vi "observacao_queued.vi"() -> ()   [LabVIEW 2012, in "Shared_160.lvlib"]
uses:
  Shared_160.lvlib
  Control 1.ctl
  System.Windows.Forms
  Global_Telescopio.vi
  Global Tabs.vi
panel:
  out "element":string
  out "size(s)":i32
  out "timeStatShutterAlert":i32
  out "sendCommandShutter":bool
  out "shutterTimeOld":i32
  out "LEAF":i32
  in  "Default":string="DEFAULT"
  out "Flag ativo DEC":bool
  out "Flag ativo AH":bool
  out "Flag de erro p/ apagar lampada":bool
  out "Cont-ShutOpen":timestamp
  out "Flag-ShutClose":bool
  out "Flag-ShutOpen":bool
  in  "erro lig":i32=3
  in  "erro des":i32=3
  in  "xxz":string
  out "Flag desligar":bool
  out "Flag ligar":bool
  out "Flag Stop":bool
  in  "AUX LAMPADA":bool
  out "Apontou":bool caption="Working Area"
  in  "AUX ABA":bool
  out "error out 5":errorcluster
  in  "error in (no error)":errorcluster
  out "AH_Destino":dbl format="%.9g"
  out "CONT DEC UTILS":i32
  out "CR DEC UTILS":i32
  out "CONT AH UTILS":i32
  out "CR AH UTILS":i32
  out "Erro PROTEC":i32=5
  out "Erro Lim":i32=5
  out "Flag Alarm":bool
  out "alarm Time":timestamp
  out "error out 4":errorcluster
  in  "Case Constant\n(See Context Help) 21":bool=TRUE
  in  "Case Constant\n(See Context Help) 19":bool=TRUE
  in  "Case Constant\n(See Context Help) 18":bool
  in  "Case Constant\n(See Context Help) 17":bool=TRUE
  in  "Case Constant\n(See Context Help) 16":bool
  in  "LedPointing":bool=TRUE
  in  "Case Constant\n(See Context Help) 15":bool
  in  "Case Constant\n(See Context Help) 14":bool=TRUE
  in  "Case Constant\n(See Context Help) 13":bool=TRUE
  in  "Case Constant\n(See Context Help) 12":bool=TRUE
  in  "Case Constant\n(See Context Help) 11":bool
  in  "Case Constant\n(See Context Help) 10":bool
  in  "Case Constant\n(See Context Help) 9":bool
  in  "Disabled":u8=2
  in  "Case Constant\n(See Context Help) 8":bool=TRUE
  in  "Case Constant\n(See Context Help) 7":bool=TRUE
  in  "Case Constant\n(See Context Help) 6":bool
  in  "Case Constant\n(See Context Help) 5":bool
  in  "TRUE=HORA\nFALSE=GRAU":bool=TRUE
  in  "Case Constant\n(See Context Help) 4":bool
  in  "Case Constant\n(See Context Help) 3":bool
  in  "Case Constant\n(See Context Help) 2":bool
  in  "Case Constant\n(See Context Help)":bool
  out "TA3":u32
  out "TA2":u32
  out "TF2":u32
  out "TF1":u32
  out "TA1":u32
  out "Tick Cupula":u32
  out "T2 3":u32
  in  "ESTADO ABRIR":string
  in  "ESTADO FECHAR":string
  out "T2 2":u32
  out "T1 2":u32
  out "T2":u32
  out "T1":u32
  out "DEC":string="00 00 00,00"
  out "Hour Angle 2":string="00 00 0,00" caption="AH"
  in  "TIMER TICK":u32
  in  "STOP":bool
  in  "News":bool
  out "AtmosferaStr":string
  in  "BtShutterClose":bool caption="DOME SHUTTER"
  out "HA obs":dbl
  out "Time to Limit":string
  in  "Clear All Messages":bool
  out "FiltroDuplo":bool
  out "ObjCentrado":bool
  out "Timeout PROT":u32
  out "LIMITE":bool
  in  "DestCUP":i16
  in  "DestAH":dbl
  in  "DestDEC":dbl
  in  "M_CUP":i32
  out "TimeoutCUP 2":u32
  out "TimeoutAH 2":u32
  out "TimeoutDEC 2":u32
  in  "Max":dbl=2300.0
  in  "Min":dbl=200.0
  out "error out":errorcluster
  out "TUBO_STAT":string
  out "CUP_STAT":string
  out "DEC_STAT":string
  out "AH_STAT":string
  out "FOCO_ENC":string
  out "DEC_ENC":string
  out "AH_ENC":string
  out "RA on Target":bool
  in  "BtOnTatget":bool
  out "Offset DEC":dbl format="%#.2f"
  out "Offset RA":dbl format="%#.2f"
  out "Mount Fine Movement":bool
  out "Mount Gross Movement":bool
  in  "follow redirects (T)":bool=TRUE
  out "header":string
  out "subarray":string[][](array[string])
  out "Draw Area 4":cluster{"Width":u32, "Height":u32}
  out "Draw Area 3":cluster{"Width":u32, "Height":u32}
  in  "sair":bool
  out "Saida Path string":string
  out "AUX EDITA RA":string caption="Name"
  out "Sideral time":string caption="ST"
  out "UT":string
  out "FLAG SET COORD":bool
  out "AUX EDITA PMDEC":string caption="Name"
  out "AUX EDITA PMRA":string caption="Name"
  out "AUX EDITA EPOCH":string caption="Name"
  out "AUX EDITA DEC":string caption="Name"
  out "AUX EDITA Name":string caption="Name"
  out "Hour Angle":string="00 00 0,00"
  in  "DECTARGET":string
  in  "AHTARGET":string
  out "Zenital angle":dbl
  out "SlideEnviromental":dbl(slide) caption="Progress ..." scale=0.0..100.0
  out "RA AUX":string
  out "EPOCH AUX":string
  out "Draw Area 2":cluster{"Width":u32, "Height":u32}
  out "SYSTEM MESSAGES":string
  out "Data Acquisition Activity":bool
  out "Auto guider Activity":bool
  out "Security Zone":bool
  out "Precess Data out-of-date":bool
  out "D...":bool
  out "C...":bool
  out "B...":bool
  out "A...":bool
  out "DEC on Target":bool
  out "Dome on Target":bool
  out "Remote User in Control":bool
  out "Air Mass":dbl
  out "Epoch":dbl
  out "Right Ascention":string="00 00 00,00"
  out "Declination":string="00 00 00,00"
  out "Azimuth":dbl
  out "Wind Chill":dbl
  out "Boolean 11":bool
  out "Wind Dir":string
  in  "Int/Ext":bool=TRUE
  out "Temperature":dbl
  out "Humidity":dbl
  out "Dew Point":dbl
  out "Wind Speed":dbl
  out "Pressure":dbl
  in  "RESTART METEOR":bool
  in  "VARIABLE \nTRACKING":bool
  out "LED VAR TRACKING":bool
  out "LED GUIDER":bool
  out "Led Chave Dome":bool
  out "LED MOUNT":bool
  in  "GUIDER":bool
  in  "DOME":bool
  in  "MOUNT":bool
  out "NAME":string
  out "DEC":string
  out "RA":string
  in  "Tab Control":T1(tab)=enum."Test Only"
  in  "IMAGE 5":bool
  out "Image":picture
  in  "PictureBox":refnum<k24>(container)
  out "Image 2":picture
  in  "IMAGE 2":bool
  out "error out 3":errorcluster
  out "error out 2":errorcluster
  in  "IMAGE 4":bool
  out "Image 4":picture
  out "pressão atm":string
  out "hum local":string
  out "Temp amb":string
  in  "IMAGE 3":bool
  out "Image 3":picture
  in  "IMAGE 6":bool
  out "Image 3a":picture
  out "C. AH":i32
  out "DOMO_ENC":string
  out "Proteção":bool
  in  "M_PROT":i32
  out "dt":u32
  out "TUBO":bool[](array[boolean])
  out "CUP":bool[](array[boolean])
  out "DEC":bool[](array[boolean])
  out "RA":bool[](array[boolean])
  in  "statCUP":i32
  in  "statAH":i32
  in  "statDEC":i32
  out "statCUP 2":i32
  out "TimeoutCUP":u32
  out "Azimute cup":u16
  out "PosCUP":i16
  out "dtAUX2":u32
  out "dtAUX3":u32
  out "PosAH":dbl
  out "PosDEC":dbl
  out "dec=":bool
  out "ah=":bool
  in  "CR AH":i32
  in  "CR DEC":i32
  out "C. DEC":i32
  in  "M_AH":i32
  in  "M_DEC":i32
  in  "Stop All":bool
  in  "Setup, Pointing & Guiding":T2(tab)=enum."POINTING"
  in  "RA Max 2":i32 min=-6 max=23
  in  "RA Min 2":i32 min=-6 max=23
  out "Erro":bool
  in  "MAG Max":dbl min=-9.0 max=100.0
  in  "MAG Min":dbl min=-9.0 max=25.0
  in  "DEC Max":i32 min=-90 max=90
  in  "DEC Min":i32 min=-90 max=90
  in  "RA Max":i32 caption="AH Max" min=-6 max=23
  in  "RA Min":i32 caption="AH Min" min=-6 max=23
  in  "Filter RA":bool
  in  "Slide old":i32
  out "Tot Linhas":i32
  in  "Open BSC":bool
  in  "Slide":dbl(slide) min=0.0 max=24.0 step=0.024 scale format="%#_3g"
  in  "EDIT":bool
  in  "Insert":bool
  out "List File":string
  in  "Upload":bool
  in  "Open":bool
  in  "Save AS":bool
  in  "Save":bool
  in  "Clear ALL":bool
  in  "SET coord":bool
  in  "Delete":bool
  in  "Multicolumn Listbox":i32[](listbox)
  out "ScaleMin":string
  out "ScaleMax":string
  out "DEC obs":dbl format="%.9f"
  out "RA obs":dbl format="%.9f"
  in  "ChkPointPrecessed":bool
  in  "Processa Centragem":bool
  out "PM_DEC":string
  out "PM_RA":string
  out "LedPointing":bool caption="Telescope Pointing"
  out "TimeoutAH":u32
  out "TimeoutDEC":u32
  out "AtualDEC":dbl format="%.9f"
  out "MeanDEC":string
  out "MeanRA":string
  in  "MAG":string
  out "Zenital Angle":string
  out "Air Mass":string
  out "Tempo Obs":string
  in  "BtPointPrecess":bool
  in  "ChkCalGlobal":bool=TRUE
  in  "ChkCalLocal":bool caption="Use Local Zero"
  in  "ChkPoinLampOFF":bool=TRUE
  in  "ChkPointRNA":bool
  in  "ChkModel":bool=TRUE
  in  "ChkWindDown":bool
  in  "ChkOpenShutter":bool
  in  "ChkDomeEnable":bool
  out "LedPointWorkArea":bool caption="Working Area"
  in  "BtTargetPoint":bool
  out "StrPointTargetDEC":string caption="Declination"
  out "StrPointTargetRA":string caption="Right Ascension"
  in  "BtPointObjClear":bool
  in  "StrPointObjPMDEC":string caption="DEC Proper Motion"
  in  "StrPointObjPMRA":string caption="RA Proper Motion"
  in  "StrPointObjName":string caption="Name"
  in  "StrPointObjEpoch":string caption="Epoch"
  in  "StrPointObjDEC":string caption="Declination"
  in  "StrPointObjRA":string caption="Right Ascension"
  out "MOV_IDX_DEC":bool
  out "MOV_IDX_AH":bool
  out "LatchDeslocDEC":dbl caption="DEC"
  out "LatchDeslocRA":dbl caption="RA"
  in  "ClearDeslocDEC":bool
  in  "ClearDeslocRA":bool
  out "DeslocDEC":dbl caption="DEC" format="%#.1f"
  out "DeslocRA":dbl caption="RA" format="%#.1f"
  in  "Delete Calagem":bool
  in  "Global":bool caption="Local"
  in  "Calagem":bool
  in  "Up HS":bool
  in  "Right HS":bool
  in  "Down HS":bool
  in  "Left HS":bool
  in  "Velocity (arcsec/sec)":i32(slide) min=0 max=600 scale=0.0..600.0
  in  "BtPrecGO":bool
  in  "BtPrecCentrar":bool
  in  "PreciseOffsetDEC":dbl caption="DEC" min=-10000.0 max=10000.0 step=1.0 format="%.3g"
  in  "PreciseOffsetRA":dbl caption="RA . cos(delta)" min=-10000.0 max=10000.0 step=1.0 format="%.3g"
  in  "Habilita Movimento":bool=TRUE
  in  "Y STAR":i32=1 min=1 max=400 step=1
  in  "X STAR":i32=1 min=1 max=400 step=1
  in  "XY CENTER":bool
  in  "Y CENTER":i32=1 min=1 max=400 step=1
  in  "X CENTER":i32=1 min=1 max=400 step=1
  in  "ClearRA":bool
  in  "ClearDEC":bool
  in  "DEC RATE":i32 min=-2000 max=2000 step=1
  in  "RA  RATE":i32 min=-2000 max=2000 step=1
  out "old":i32 min=0 max=360
  in  "Velocity":dbl(slide)=0.01 caption="(max = 65535 u/s)" min=0.01 max=100.0 step=0.01 scale=0.0..100.0
  in  "focusHome":bool
  out "focusStatus":string="            Focus Status"
  out "focuAlarm":bool caption="Motor temp."
  out "focusHoming":bool caption="Homing"
  out "focusMoving":bool caption="Moving"
  out "focusConnected":bool
  out "focusInitialized":bool
  in  "SetDefaultFocus":bool
  out "Foco":dbl(slide) caption="1" scale=0.0..50000.0
  in  "Setpoint":dbl=200.0 caption="Target" min=200.0 max=2300.0 step=1.0
  in  "GO":bool
  in  "Focus +":bool caption="Focus Out (+)"
  in  "Focus -":bool caption="Focus In (-)"
  in  "New Angle":string="    0.0"
  out "Default Angle":string="      0.00"
  in  "SetRotatorDefAngle":bool
  in  "Set Rotator Angle":bool
  out "Rotator Angle":string="  0.00" caption="for  GUIDING"
  out "StatShutterFile":string
  out "Command":string
  in  "CCW":bool
  out "RefreshShutterState":bool
  in  "BtParavStop":bool
  in  "BtParavUp":bool
  in  "BtParavDown":bool
  out "LedShutter":bool
  out "TimeoutTrap":u32
  out "StatShutter":string caption="Control State"
  in  "BtShutClose":bool
  in  "BtShutOpen":bool
  out "StatDome":string caption="Control State"
  in  "BtDomeSTOP":bool
  in  "BtDomeGO":bool caption="DOME"
  in  "DomeNewPos":i32=30 caption="New Position" min=0 max=360
  out "PosCup":i16 caption="Position"
  in  "CW":bool
  out "LED ACTION":bool
  out "LED MODE":bool
  in  "ACTION":bool
  in  "MODE":bool
  in  "Default Met":bool=TRUE
  in  "PROTEÇÃO":bool
  in  "STOP":bool
  in  "Enable Centragem":bool=TRUE
  in  "GO":bool
  in  "StrPointObjDEC 2":string caption="DEC"
  in  "StrPointObjRA 2":string caption="AH"
  out "MOVING":bool
  in  "FLAT-FIELD":bool
  in  "BtUtilPark":bool
  in  "ECASS":bool
  in  "BtUtilZenith":bool
  in  "TabInstrumento":T3(tab)=enum."Cam 1"
  out "Posição Rede":i32=10 caption="Largura da Fenda" min=10 max=5000 step=1
  in  "HomePrisma":T4 caption="DOME"
  in  "HomeEspelho":T4 caption="DOME"
  in  "HomeFenda":T4 caption="DOME"
  in  "IronArc":bool=TRUE
  out "Boolean":bool
  out "Largura da Fenda 2":dbl=10.0 caption="Largura da Fenda" min=10.0 max=5000.0 step=1.0
  in  "Prisma das Lâmpadas":bool
  out "Position":string
  in  "Largura da Fenda":dbl=10.0 min=10.0 max=5000.0 step=1.0
  in  "Go Largura da Fenda":bool caption="DOME"
  in  "Angulo da rede de difração":i32=10 caption="Ângulo da Rede" min=10 max=99989 step=1
  in  "Go Angulo de Difração":bool caption="DOME"
  in  "Incand":bool=TRUE
  in  "Neon":bool=TRUE
  in  "Cathode":bool=TRUE
  out "Ang. Fenda":dbl
  in  "Go_Coudé":bool
  in  "Radio Buttons":enum32{"Azul", "Visível", "Vermelho"}(radio)
  out "EndTime":u32
  out "ledAzul":bool
  out "ledVisivel":bool
  out "ledVermelho":bool
  in  "MENSAGEM":string="EM MOVIMENTO"
  out "MENSAGEM 2":string="EM MOVIMENTO"
  out "#2":bool
  out "#3":bool
  out "#4":bool
  out "PosSecundario":bool
  out "Cjto_3":bool
  out "EspAtual":string
  out "parou":bool
  out "parou 2":bool
  out "Posição Espelho":dbl=10.0 caption="Largura da Fenda" min=10.0 max=5000.0 step=1.0
  out "parou 3":bool
  out "Output Message":string
  in  "stopEcass":bool
  out "SlideEcass":u8(slide) caption="Espelho movendo..." max=100 scale=0.0..100.0
  out "LedRep":bool
  out "LedCal":bool
  in  "Sent_EspLampCass":bool
  out "LedHe":bool
  out "LedNe":bool
  in  "He-Ar":bool
  in  "Ne":bool
  in  "stopCam1":bool
  out "SlideCam1":u8(slide) caption="Espelho movendo..." max=100 scale=0.0..100.0
  out "LedRepCam1":bool
  out "LedCalCam1":bool
  in  "Sent_EspDesvFeixe":bool
  in  "Go_filtro":bool
  in  "Filtro":string(combo)
  in  "Mover/Parar":bool
  out "Recuar":bool
  in  "Sentido":bool=TRUE
  in  "Velocidade":bool
  out "Rapido":bool
  out "Lento":bool
  out "Avancar":bool
  out "Comando":string
  in  "Mensage Alarme":string="To light up close the Shutter !"
  out "CoudeSel":bool
  in  "Coude":bool
  in  "BtCalFlatField":bool
  in  "ChkCalLamp4":bool
  in  "ChkCalLamp3":bool
  in  "ChkCalLamp2":bool
  in  "ChkCalLamp1":bool
  in  "BtCalTurnOff":bool
  in  "BtCalTurnOn":bool
  out "StrongSel":bool
  out "MediumSel":bool
  out "WeakSel":bool
  in  "Strong":bool
  in  "Medium":bool
  in  "Weak":bool
  # "TELESCOPE CONTROL SYSTEM\nPICO DOS DIAS OBSERVATORY"
  # "Status Information"
  # "System Positions"
  # "Environmental Status"
  # "EXT"
  # "INT"
  # "mBar"
  # "o"
  # "C"
  # "Km/h"
  # "%"
  # "o"
  # "o"
  # "C"
  # "C"
  # "CLOUSURE LIMITS"
  # "Wind Speed            >  70 Km/h\nRelative Humidity    >  97 %\nInternal Dewpoint  <  0.5  C\nExternal Dewpoint <  1.0  C"
  # "OBJECT"
  # "TRACKING ENABLE"
  # "%"
  # "Conector 4"
  # "Conector 3"
  # "ALARME\nATENÇÃO\nERROS\nOCUPADO"
  # "Proteção\n\nTracking\nVar_Track"
  # "Rapido\nLigeiro\nFino\nRun"
  # "Motor\nIDX_Rdy\nManual"
  # "BSC FILTERS"
  # "LIST FILE"
  # "OBJECT INPUT"
  # "TARGET"
  # "OPTIONS"
  # "MANUAL OFFSET"
  # "PRECISE OFFSET"
  # "N"
  # "E"
  # "W"
  # "arcsec"
  # "arcsec"
  # "S"
  # "DISPLACEMENT"
  # "CALAGEM"
  # "PODE NÃO FUNCIONAR CORRETAMENTE!"
  # "STAR CENTERING"
  # "VAR. TRACKING"
  # "AUTO-GUIDER COORDINATES"
  # "1) Entrar X e Y do cursor do Autoguider correspondente à posição de centragem nas entradas X CENTER e Y CENTER. \n2) Após apontamento, entrar em X STAR e Y STAR os valores de X e Y do Autoguider com o \"Guide Box\" sobre o objeto apontado. \n3) Clicar em MOVE STAR TO CENTER."
  # "May take many\ntens of seconds"
  # "(instrument)"
  # "Continuous Movement"
  # "ATENÇÃO:\nO Rotator ainda não está integrado ao sistema de controle e como sua posição afeta a guiagem, sempre que o rotator for girado manualmente é necessário digitar o valor de sua nova posição no controle \"New Angle\" e pressionar \"SET NEW\".\n\nPressionar \"SET NEW\" ou \"SET DEFAULT\" não gira o rotator!"
  # "ROTATION"
  # "SHUTTER"
  # "WINDSCREEN"
  # "Covers"
  # "FIXED POSITIONS"
  # "Acquisition System\nON TARGET command"
  # "Select one Mirrror"
  # "Mirror #2"
  # "Mirror #3"
  # "Mirrors Drivers"
  # "Lâmpadas de Calibração"
  # "Espelho das Lâmpadas de Calibração"
  # "Posição"
  # "Repouso"
  # "Ativo"
  # "LIGA"
  # "LIGA"
  # "DESL."
  # "DESL."
  # "Espelho do Eucalyptus"
  # "Roda de filtros"
  # "Posição"
  # "Repouso"
  # "Ativo"
  # "Espelho de Campo"
  # "Recuar"
  # "Avançar"
  # "Rápido"
  # "Lento"
  # "CALIBRATION LAMPS"
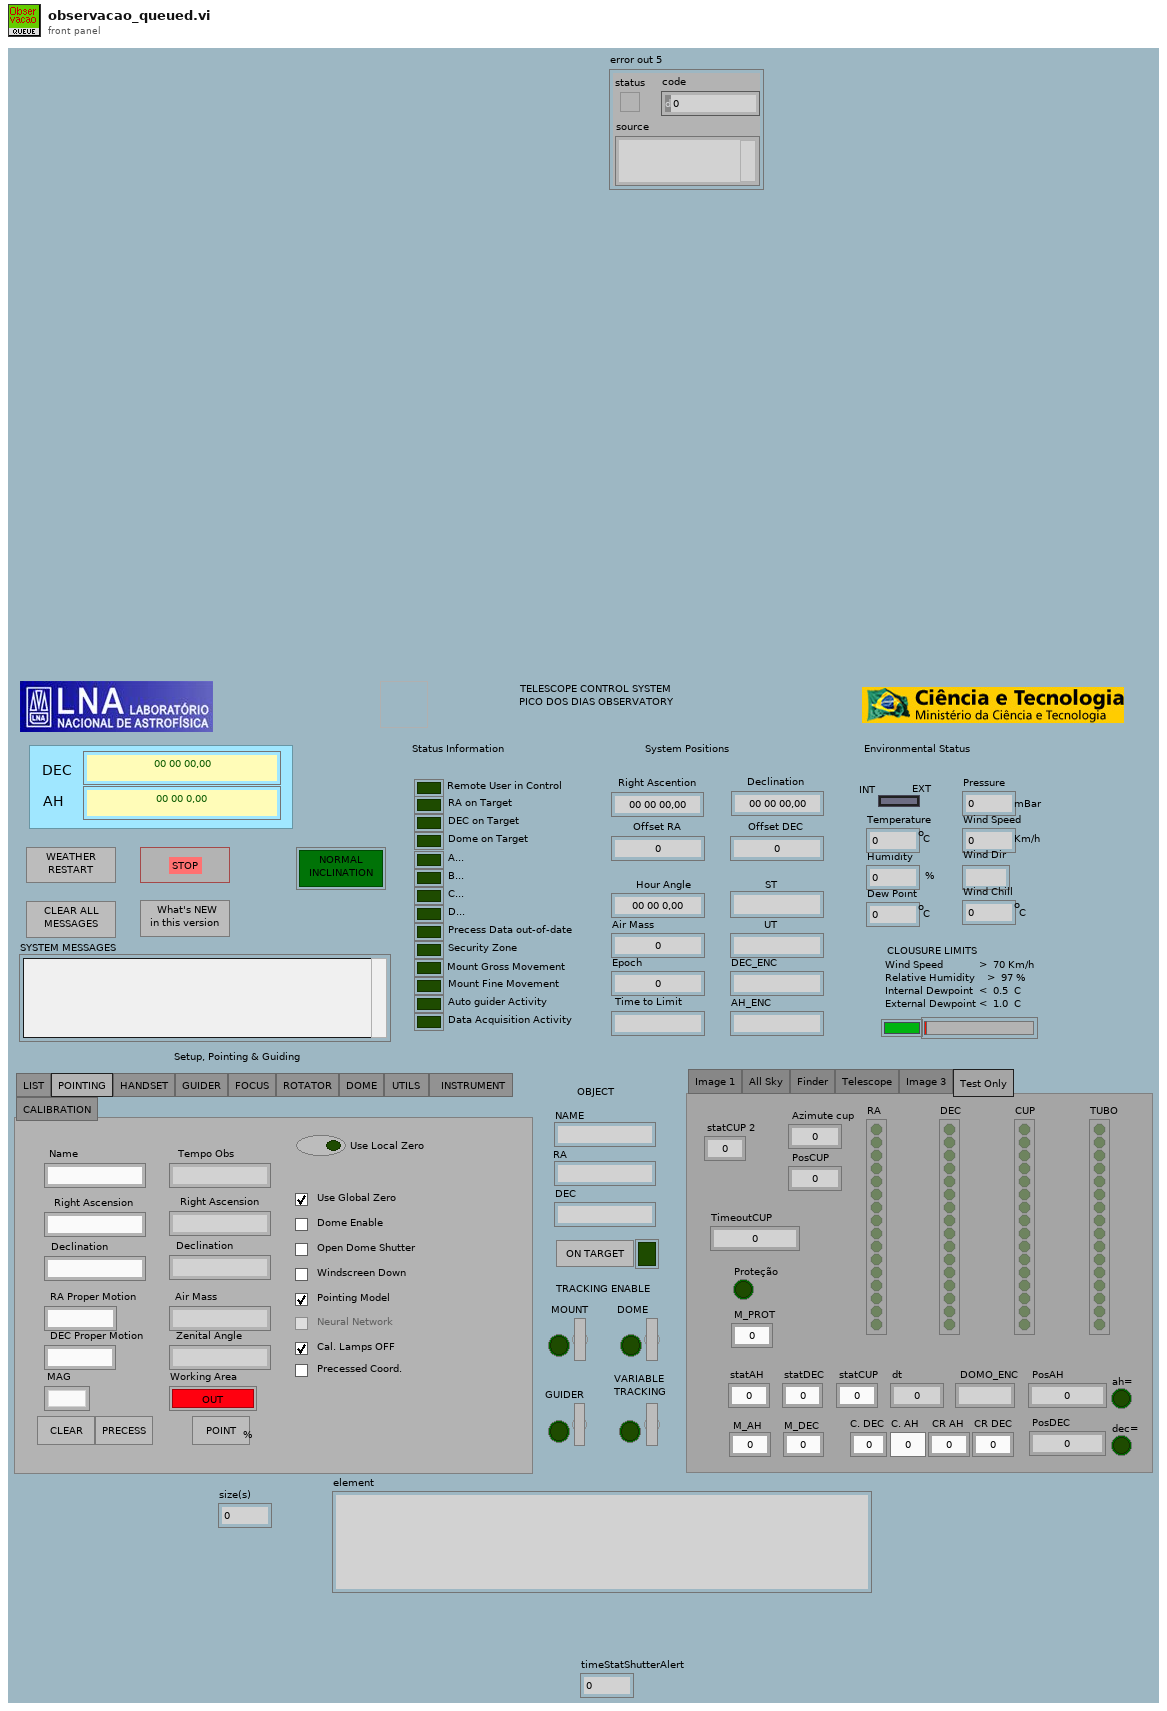
[diagram p1: front panel]
types:
  T1 = enum32{"Image 1", "All Sky", "Finder", "Telescope", "Image 3", "Test Only"}
  T2 = enum32{"LIST", "POINTING", "HANDSET", "GUIDER", "FOCUS", "ROTATOR", "DOME", "UTILS ", " INSTRUMENT ", "CALIBRATION"}
  T3 = enum32{"Coude", "Casseg.", "Eucalyp.", "Cam 1", "Cam 2", "Cam IV.", "Polarim.", "Fotrap"}
  T4 = typedef "Control 1.ctl" = bool
  T5 = enum8{"Enabled", "Disabled", "Disabled and Grayed Out"}
  T6 = enum32{"Page Enabled", "Page Disabled", "Page Disabled & Grayed"}
  T7 = enum16{"open", "replace", "create", "open or create", "replace or create", "replace or create with confirmation"}
  T8 = enum16{"open", "open or create", "create or replace", "create"}
  T9 = enum16{"open", "open or create", "create or replace", "create", "open (read only)"}
  T10 = typedef "LVRemotePanelConnectionsTypeDef.ctl" = cluster{"VI Name":string, "Remote":string, "UserName":string, "Port":i32, "Status":enum32{"Viewing", "Waiting For Control", "Controlling"}, "Create Time":timestamp, "Status Time":timestamp, "Control End Time":timestamp}[]
  T11 = cluster{"absolute":bool, "alarm":bool, "cmd":cluster{"clientId":dbl, "clientTransactionId":dbl, "clientName":string, "action":string}, "connected":bool, "controller":string, "device":string, "error":string, "homing":bool, "initialized":bool, "isMoving":bool, "maxSpeed":dbl, "maxStep":dbl, "position":dbl, "tempComp":bool, "tempCompAvailable":bool, "temperature":dbl, "timestamp":dbl}
  T12 = cluster{"clientId":dbl, "clientTransactionId":dbl, "clientName":string, "action":string}
  T13 = cluster{"left":i16, "top":i16, "right":i16, "bottom":i16}
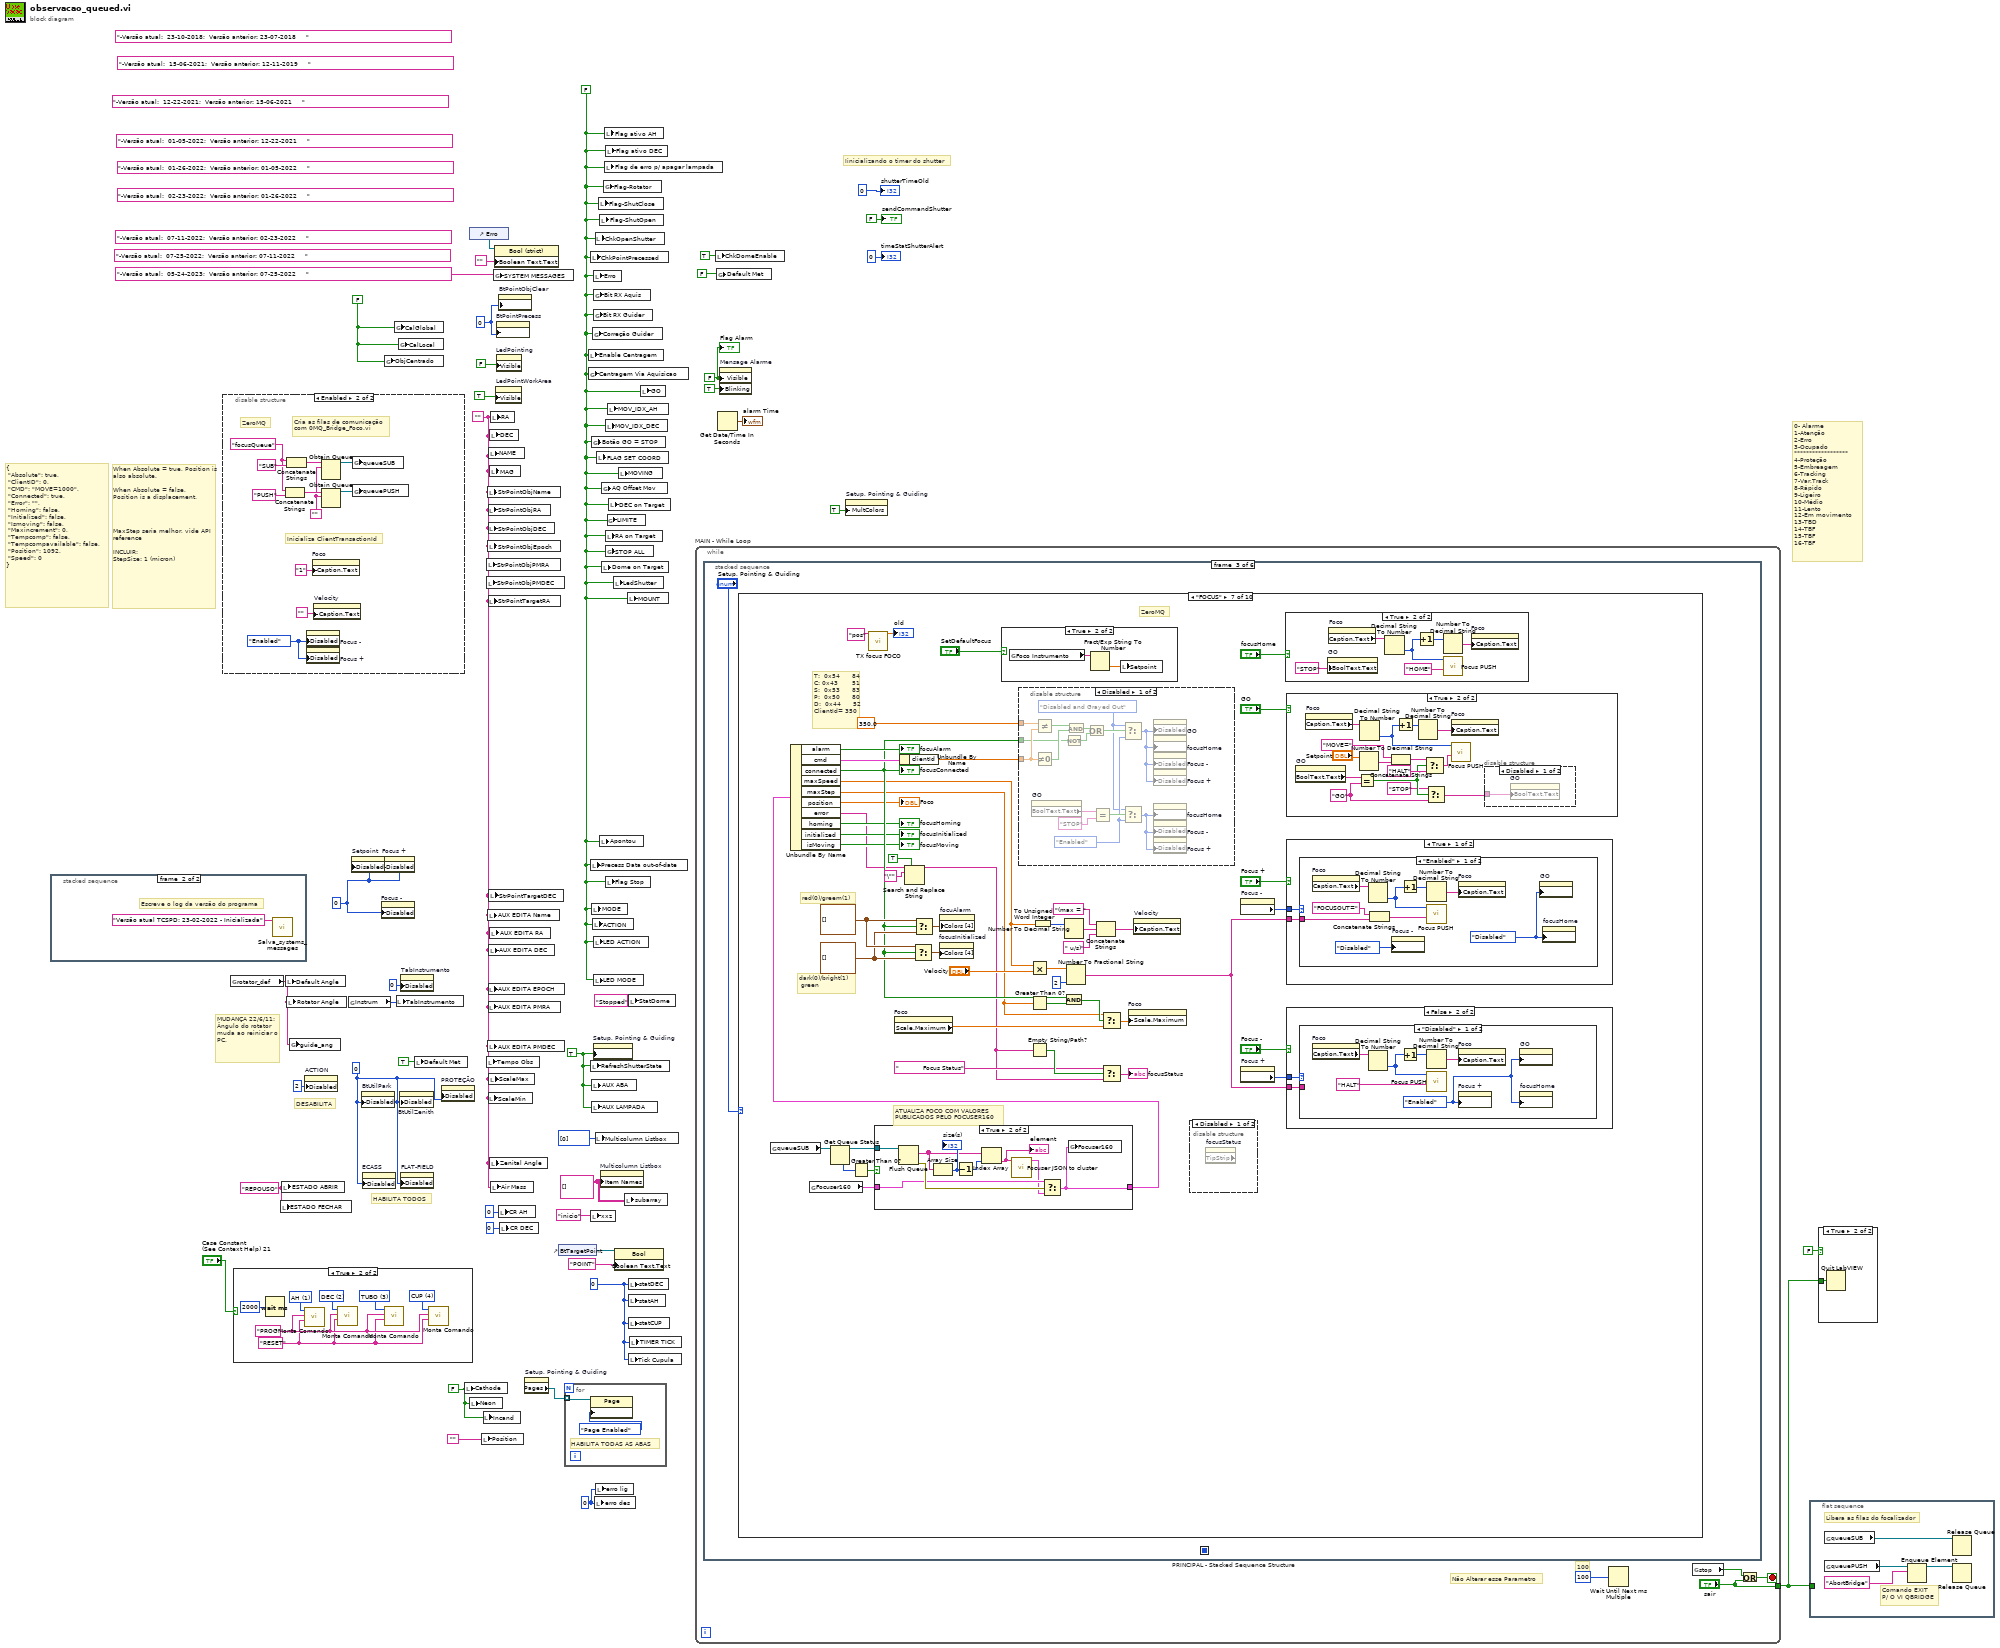
[diagram p0: block diagram]
diagram:
  (unwired) "-Versão atual:  07-25-2022;  Versão anterior: 07-11-2022     " ("SYSTEM MESSAGES")
  (unwired) "-Versão atual:  07-11-2022;  Versão anterior: 02-23-2022     " ("SYSTEM MESSAGES")
  (unwired) "-Versão atual:  02-23-2022;  Versão anterior: 01-26-2022     " ("SYSTEM MESSAGES")
  (unwired) "-Versão atual:  01-26-2022;  Versão anterior: 01-05-2022     " ("SYSTEM MESSAGES")
  (unwired) "-Versão atual:  01-05-2022;  Versão anterior: 12-22-2021     " ("SYSTEM MESSAGES")
  (unwired) "-Versão atual:  12-22-2021;  Versão anterior: 15-06-2021     " ("SYSTEM MESSAGES")
  (unwired) "-Versão atual:  15-06-2021;  Versão anterior: 12-11-2019     " ("SYSTEM MESSAGES")
  w10 = 0
  w11 = 0 ("erro des")
  w17 = FALSE ("Visible")
  w21 = FALSE ("ThAr")
  w23 = "REPOUSO" ("y")
  (unwired) "-Versão atual:  23-10-2018;  Versão anterior: 23-07-2018     " ("SYSTEM MESSAGES")
  w35 = u8 0 ("Disabled")
  w13 = TRUE ("Page Selector Visible")
  w38 = FALSE ("Set aux")
  w39 = u8 0 ("Disabled")
  w22 = 0 ("estado")
  w30 = ""
  w40 = string[][] [] ("Item Names")
  w9 = FALSE ("Set aux")
  # "When Absolute = true, Position is also absolute.\n\nWhen Absolute = false,\nPosition is a displacement.\n\n\n\n\nMaxStep seria melhor, vide API reference\n\nINCLUIR:\nStepSize: 1 (micron)"
  # "{\n \"Absolute\": true,\n \"ClientID\": 0,\n \"CMD\": \"MOVE=1000\",\n \"Connected\": true,\n \"Error\": \"\",\n \"Homing\": false,\n \"Initialized\": false,\n \"Ismoving\": false,\n \"Maxincrement\": 0,\n \"Tempcomp\": false,\n \"Tempcompavailable\": false,\n \"Position\": 1092,\n \"Speed\": 0\n}"
  # "Iinicializando o timer do shutter"
  # "DESABILITA"
  # "MUDANÇA 22/6/11:\nÂngulo do rotator muda ao reiniciar o PC."
  # "HABILITA TODOS"
  # "0- Alarme\n1-Atenção\n2-Erro\n3-Ocupado\n******************\n4-Proteção\n5-Embreagem\n6-Tracking\n7-Var.Track\n8-Rápido\n9-Ligeiro\n10-Médio\n11-Lento\n12-Em movimento\n13-TBD\n14-TBF\n15-TBF\n16-TBF"
  n1 = stacked-sequence {
    frame #0 {
      # "Escreve o log da estação\nmetereologica"
      # "Alterado 11/12/2012 est.\nmeteorológica"
      n2 = call "Teste_Read_Meteorologica.vi"() -> ()  [unwired: 2 in, 1 out]
    }
    frame #1 {
      # "Escreve o log da versão do programa"
      n3 = call "Salva_systems_messages.vi"("Mensagem"="Versão atual TCSPD: 23-02-2022 - Inicializada" ("message")) -> ()  [unwired: 5 in]
    }
  }
  n4 = disable-structure shown="Enabled" {
    frame Disabled {
      w46 = u8 1 ("OutOfRngActMin")
      w48 = FALSE ("Set aux")
      # "ZeroMQ"
      # "iniciação aba focus"
      n5 = stacked-sequence {
        frame #0 {
          n6 = global write "Global Tabs.vi" "Off-foc"(0.0 ("Offset")) -> ()
        }
        frame #1 {
          n7 = call "TX focus FOCO.vi"("Comando"="pos") -> ("pos (deg)"=w52:dbl)  [unwired: 12 in, 2 out]
          n8 = global write "Global_Telescopio.vi" "Foco"(w52) -> ()
          n9 = local write "Foco"(w52) -> ()
          n10 = local write "Setpoint"(w52) -> ()
        }
      }
      n11 = property on="Foco" class="Slide (strict)"("Scale.Range:Minimum"="Min", "Scale.Range:Maximum"="Max") -> ()  [unwired: 2 in, 2 out]
      n12 = property on="Setpoint" class="DigNum (strict)"("Data Entry Limits:Minimum"="Min", "Data Entry Limits:Maximum"="Max", "Response to Value Outside Limits:Maximum"=w46, "Response to Value Outside Limits:Minimum"=w46) -> ()  [unwired: 2 in, 2 out]
      n13 = control-ref of="GO"() -> (w50:refnum<vi>)
      n14 = property class="Bool"(reference=w50, "Boolean Text.Text"="GO") -> ()  [unwired: 1 in, 2 out]
      n15 = local write "Focus +"(w48) -> ()
      n16 = local write "Focus -"(w48) -> ()
    }
    frame Enabled {
      w54 = T5."Enabled" ("Disabled")
      w59 = "focusQueue" ("string")
      w60 = ""
      # "Inicializa ClientTransactionId"
      # "Cria as filas de comunicação\ncom 0MQ_Bridge_Foco.vi"
      # "ZeroMQ"
      n17 = Concatenate Strings(w59, "PUSH" ("string")) -> (w62:string)
      n18 = Concatenate Strings(w59, "SUB" ("string")) -> (w61:string)
      n19 = property on="Focus -" class="Bool (strict)"("Disabled"=w54) -> ()  [unwired: 2 in, 2 out]
      n20 = property on="Focus +" class="Bool (strict)"("Disabled"=w54) -> ()  [unwired: 2 in, 2 out]
      n21 = property on="Foco" class="Slide (strict)"("Caption.Text"="1") -> ()  [unwired: 2 in, 2 out]
      n22 = property on="Velocity" class="Slide (strict)"("Caption.Text"="") -> ()  [unwired: 2 in, 2 out]
      n23 = Obtain Queue(name (unnamed)=w61, element data type=w60) -> (queue out=w58:refnum<queue>)  [unwired: 3 in, 2 out]
      n24 = Obtain Queue(name (unnamed)=w62, element data type=w60) -> (queue out=w57:refnum<queue>)  [unwired: 3 in, 2 out]
      n25 = global write "Global_Telescopio.vi" "queueSUB"(w58) -> ()
      n26 = global write "Global_Telescopio.vi" "queuePUSH"(w57) -> ()
    }
  }
  n27 = global read "Global_Telescopio.vi" "rotator_def"() -> (w26:string)
  n28 = case shown="True" "Case Constant\n(See Context Help) 21" {
    frame False {
    }
    frame True {
      w67 = u16 4 items=["ZERO", "AH", "DEC", "TUBO", "CUP"] ("Controlador")
      w68 = u16 3 items=["ZERO", "AH", "DEC", "TUBO", "CUP"] ("Controlador")
      w70 = u16 2 items=["ZERO", "AH", "DEC", "TUBO", "CUP"] ("Controlador")
      w66 = "PROG" ("Comando")
      w65 = "RESET" ("Comando")
      w71 = u16 1 items=["ZERO", "AH", "DEC", "TUBO", "CUP"] ("Controlador")
      n29 = Wait (ms)(milliseconds to wait=u32 2000) -> ()  [unwired: 1 out]
      n30 = call "Monta Comando.vi"("Comando"=w65, "Dispositivo"=w66, "Controlador"=w71) -> ()  [unwired: 4 in, 3 out]
      n31 = call "Monta Comando.vi"("Comando"=w65, "Dispositivo"=w66, "Controlador"=w70) -> ()  [unwired: 4 in, 3 out]
      n32 = call "Monta Comando.vi"("Comando"=w65, "Dispositivo"=w66, "Controlador"=w68) -> ()  [unwired: 4 in, 3 out]
      n33 = call "Monta Comando.vi"("Comando"=w65, "Dispositivo"=w66, "Controlador"=w67) -> ()  [unwired: 4 in, 3 out]
    }
  }
  n34 = local write "ESTADO FECHAR"(w23) -> ()
  n35 = local write "ESTADO ABRIR"(w23) -> ()
  n36 = local write "Default Angle"(w26) -> ()
  n37 = local write "Rotator Angle"(w26) -> ()
  n38 = global write "Global_Telescopio.vi" "guide_ang"(w26) -> ()
  n39 = property on="ACTION" class="Bool (strict)"("Disabled"=u8 2) -> ()  [unwired: 2 in, 2 out]
  n40 = global read "Global_Telescopio.vi" "Instrum"() -> (w33:u16)
  n41 = property on="Setpoint" class="DigNum (strict)"("Disabled"=w39) -> ()  [unwired: 2 in, 2 out]
  n42 = property on="BtUtilPark" class="Bool (strict)"("Disabled"=w35) -> ()  [unwired: 2 in, 2 out]
  n43 = property on="ECASS" class="Bool (strict)"("Disabled"=w35) -> ()  [unwired: 2 in, 2 out]
  n44 = property on="Focus +" class="Bool (strict)"("Disabled"=w39) -> ()  [unwired: 2 in, 2 out]
  n45 = property on="Focus -" class="Bool (strict)"("Disabled"=w39) -> ()  [unwired: 2 in, 2 out]
  n46 = global write "Global_Telescopio.vi" "ObjCentrado"(w38) -> ()
  n47 = global write "Global_Telescopio.vi" "CalGlobal"(w38) -> ()
  n48 = local write "TabInstrumento"(w33) -> ()
  n49 = global write "Global_Telescopio.vi" "CalLocal"(w38) -> ()
  n50 = property on="BtUtilZenith" class="Bool (strict)"("Disabled"=w35) -> ()  [unwired: 2 in, 2 out]
  n51 = property on="TabInstrumento" class="TabCtl (strict)"("Disabled"=u8 0) -> ()  [unwired: 2 in, 2 out]
  n52 = property on="FLAT-FIELD" class="Bool (strict)"("Disabled"=w35) -> ()  [unwired: 2 in, 2 out]
  n53 = local write "Default Met"(TRUE ("Default Met")) -> ()
  n54 = property on="PROTEÇÃO" class="Bool (strict)"("Disabled"=w35) -> ()  [unwired: 2 in, 2 out]
  n55 = local write "Cathode"(w21) -> ()
  n56 = control-ref of="Erro"() -> (w31:refnum<vi>)
  n57 = local write "Neon"(w21) -> ()
  n58 = local write "Position"("") -> ()
  n59 = local write "Incand"(w21) -> ()
  n60 = local write "StrPointObjPMRA"(w30) -> ()
  n61 = local write "StrPointObjPMDEC"(w30) -> ()
  n62 = local write "Tempo Obs"(w30) -> ()
  n63 = local write "StrPointObjName"(w30) -> ()
  n64 = local write "StrPointObjEpoch"(w30) -> ()
  n65 = local write "AUX EDITA Name"(w30) -> ()
  n66 = local write "AUX EDITA PMDEC"(w30) -> ()
  n67 = local write "StrPointObjRA"(w30) -> ()
  n68 = local write "StrPointObjDEC"(w30) -> ()
  n69 = local write "StrPointTargetRA"(w30) -> ()
  n70 = local write "AUX EDITA EPOCH"(w30) -> ()
  n71 = local write "AUX EDITA PMRA"(w30) -> ()
  n72 = local write "ScaleMin"(w30) -> ()
  n73 = local write "NAME"(w30) -> ()
  n74 = local write "StrPointTargetDEC"(w30) -> ()
  n75 = local write "AUX EDITA DEC"(w30) -> ()
  n76 = local write "ScaleMax"(w30) -> ()
  n77 = local write "MAG"(w30) -> ()
  n78 = local write "AUX EDITA RA"(w30) -> ()
  n79 = local write "Zenital Angle"(w30) -> ()
  n80 = local write "DEC"(w30) -> ()
  n81 = local write "RA"(w30) -> ()
  n82 = local write "Air Mass"(w30) -> ()
  n83 = global write "Global_Telescopio.vi" "SYSTEM MESSAGES"("-Versão atual:  05-24-2023;  Versão anterior: 07-25-2022     " ("SYSTEM MESSAGES")) -> ()
  n84 = property class="Bool (strict)"(reference=w31, "Boolean Text.Text"="") -> ()  [unwired: 1 in, 2 out]
  n85 = property on="LedPointWorkArea" class="Bool (strict)"("Visible"=TRUE ("GUIDING")) -> ()  [unwired: 2 in, 2 out]
  n86 = property on="BtPointPrecess" class="Bool"("DisabledEnum"=w10) -> ()  [unwired: 2 in, 2 out]
  n87 = property on="LedPointing" class="Bool (strict)"("Visible"=FALSE ("Set aux")) -> ()  [unwired: 2 in, 2 out]
  n88 = property on="BtPointObjClear" class="Bool"("DisabledEnum"=w10) -> ()  [unwired: 2 in, 2 out]
  n89 = local write "CR AH"(0 ("CR AH")) -> ()
  n90 = local write "CR DEC"(0 ("CR DEC")) -> ()
  n91 = property on="Setup, Pointing & Guiding" class="TabCtl (strict)"() -> ("Pages"=w36:refnum<vi>[])  [unwired: 2 in, 2 out]
  n92 = control-ref of="BtTargetPoint"() -> (w42:refnum<vi>)
  n93 = for {
    tunnel: w36 -> [w73] mode=indexing
    # "HABILITA TODAS AS ABAS"
    n94 = property class="Page"(reference=w73, "Page Enabled State"=T6."Page Enabled") -> ()  [unwired: 1 in, 2 out]
  }
  n95 = local write "Enable Centragem"(w9) -> ()
  n96 = global write "Global_Telescopio.vi" "Centragem Via Aquisicao"(w9) -> ()
  n97 = local write "ChkPointPrecessed"(w9) -> ()
  n98 = local write "Precess Data out-of-date"(w9) -> ()
  n99 = local write "RefreshShutterState"(w13) -> ()
  n100 = local write "xxz"("inicio") -> ()
  n101 = global write "Global_Telescopio.vi" "Botão GO = STOP"(w9) -> ()
  n102 = local write "MODE"(w9) -> ()
  n103 = local write "AUX ABA"(w13) -> ()
  n104 = local write "AUX LAMPADA"(w13) -> ()
  n105 = global write "Global_Telescopio.vi" "Correção Guider"(w9) -> ()
  n106 = local write "ACTION"(w9) -> ()
  n107 = global write "Global_Telescopio.vi" "Bit RX Guider"(w9) -> ()
  n108 = local write "LED ACTION"(w9) -> ()
  n109 = local write "LED MODE"(w9) -> ()
  n110 = property on="Setup, Pointing & Guiding" class="TabCtl (strict)"("Page Selector Visible"=w13) -> ()  [unwired: 2 in, 2 out]
  n111 = local write "Erro"(w9) -> ()
  n112 = global write "Global_Telescopio.vi" "Bit RX Aquis"(w9) -> ()
  n113 = local write "erro des"(w11) -> ()
  n114 = local write "ChkOpenShutter"(w9) -> ()
  n115 = local write "Multicolumn Listbox"(i32[] [0] ("Multicolumn Listbox")) -> ()
  n116 = local write "erro lig"(w11) -> ()
  n117 = local write "FLAG SET COORD"(w9) -> ()
  n118 = local write "Flag-ShutClose"(w9) -> ()
  n119 = local write "Flag-ShutOpen"(w9) -> ()
  n120 = local write "Apontou"(w9) -> ()
  n121 = property on="Multicolumn Listbox" class="MCListbox (strict)"("Item Names"=w40) -> ()  [unwired: 2 in, 2 out]
  n122 = global write "Global_Telescopio.vi" "AQ Offset Mov"(w9) -> ()
  n123 = local write "Dome on Target"(w9) -> ()
  n124 = global write "Global_Telescopio.vi" "Flag-Rotator"(w9) -> ()
  n125 = local write "Flag ativo AH"(w9) -> ()
  n126 = local write "Flag de erro p/ apagar lampada"(w9) -> ()
  n127 = local write "MOV_IDX_DEC"(w9) -> ()
  n128 = local write "RA on Target"(w9) -> ()
  n129 = global write "Global_Telescopio.vi" "STOP ALL"(w9) -> ()
  n130 = local write "Flag Stop"(w9) -> ()
  n131 = local write "Flag ativo DEC"(w9) -> ()
  n132 = global write "Global_Telescopio.vi" "LIMITE"(w9) -> ()
  n133 = local write "MOV_IDX_AH"(w9) -> ()
  n134 = local write "DEC on Target"(w9) -> ()
  n135 = local write "LedShutter"(w9) -> ()
  n136 = property class="Bool"(reference=w42, "Boolean Text.Text"="POINT") -> ()  [unwired: 1 in, 2 out]
  n137 = local write "MOVING"(w9) -> ()
  n138 = local write "subarray"(w40) -> ()
  n139 = local write "MOUNT"(w9) -> ()
  n140 = local write "Tick Cupula"(w22) -> ()
  n141 = local write "StatDome"("Stopped" ("Status")) -> ()
  n142 = local write "statDEC"(w22) -> ()
  n143 = local write "statAH"(w22) -> ()
  n144 = local write "statCUP"(w22) -> ()
  n145 = local write "TIMER TICK"(w22) -> ()
  n146 = local write "GO"(w9) -> ()
  n147 = while "MAIN - While Loop" {
    tunnel: ["sair"] -> w1
    stop <- w76 stop-if-true
    # "100"
    # "Não Alterar esse Parametro"
    n148 = stacked-sequence "PRINCIPAL - Stacked Sequence Structure" {
      seq-local: [w81 _ _ _ _ _] -> [_ w84 _ _ _ w4136]
      frame #0 {
        # "CLIENTE REMOTO"
        # "Verifica se Existe Cliente Remoto Conectado"
        n149 = invoke class="VI" method="RP.Client Connections"() -> ("Connections"=w82:T10, "Controller"=w80:i32)  [unwired: 5 in, 3 out]
        n150 = Equal?(x=w80, y=0) -> (x = y?=→"Remote User in Control":bool)
        n151 = global write "Global_Telescopio.vi" "Controller Rem/Loc"(w80) -> ()
        n152 = global write "Global_Telescopio.vi" "Dados do Computador Remoto Conectado"(w82) -> ()
        n153 = Tick Count (ms)() -> (millisecond timer value=w81:u32)
      }
      frame #1 {
        # "ACOES CONTINUAS"
        # "Cálculos Continuos / Monitoração Continua"
        n154 = stacked-sequence "MONITORACAO - Stacked Sequence Structure" {
          tunnel: w84 -> [_ _ _ w457 _ _ _ _ _ _ _ _ _ _ _ _]
          frame #0 {
            w111 = u16 3 items=["ZERO", "AH", "DEC", "TUBO", "CUP", "CASS", "COUDE"] ("Controlador")
            w119 = u16 4 items=["ZERO", "AH", "DEC", "TUBO", "CUP", "CASS", "COUDE"] ("Controlador")
            w120 = u16 2 items=["ZERO", "AH", "DEC", "TUBO", "CUP", "CASS", "COUDE"] ("Controlador")
            w123 = u16 1 items=["ZERO", "AH", "DEC", "TUBO", "CUP", "CASS", "COUDE"] ("Controlador")
            # "Monitora o programa para enviar comando\ntrapeira parar após 40s"
            # "PROCESSO LE ENCODERS"
            # "Colocar neste frame a leitura de status dos outros controladores"
            # "LEITURA STATUS DOS CONTROLADORES"
            n155 = disable-structure shown="Disabled" {
              frame Disabled {
                # "Grava o valor do foco \natual a cada minuto"
                n156 = Get Date/Time In Seconds() -> (seconds since 1Jan1904=w129:timestamp)
                n157 = Format Date/Time String(time format string (%c)="%S", seconds (now)=w129) -> (date/time string=w128:string)  [unwired: 1 in]
                n158 = Equal?(x=w128, y="00") -> (x = y?=w126:bool)
                n159 = case shown="True" w126 {
                  frame False {
                  }
                  frame True {
                    n160 = local read "Foco"() -> (w133:dbl)
                    n161 = Number To Decimal String(number=w133) -> (decimal integer string=w132:string)  [unwired: 1 in]
                    n162 = call "Log_Foco.vi"("command"=" ", "focValue"=w132, "pathLogFocoString"="C:\\TCS\\LOG\\FOCO\\") -> ()  [unwired: 6 in]
                  }
                }
              }
              frame Enabled {
              }
            }
            n163 = case shown="False" "Case Constant\n(See Context Help)" {
              selector: "Case Constant\n(See Context Help)" -> [_ w220]
              tunnel: [w219 w220] -> w121
              tunnel: w120 -> [w218 _]
              tunnel: [w217 _] -> w122
              tunnel: [w216 _] -> w93
              tunnel: [w215 _] -> w106
              frame False {
                n164 = call "Get Status Controlador.vi"("Controlador"=w218) -> ("Status"=w215:string, "Parametros"=w217:string, "Bits Status"=w216:bool[], "Erro comunicação"=w219:bool)
              }
              frame True {
              }
            }
            "DEC_STAT" <- w106
            "DEC" <- w93
            n165 = case shown="False" "Case Constant\n(See Context Help)" {
              selector: "Case Constant\n(See Context Help)" -> [_ w214]
              tunnel: [w213 w214] -> w118
              tunnel: w119 -> [w212 _]
              tunnel: [w211 _] -> w117
              tunnel: [w210 _] -> w103
              tunnel: [w209 _] -> w105
              frame False {
                n166 = call "Get Status Controlador.vi"("Controlador"=w212) -> ("Status"=w209:string, "Parametros"=w211:string, "Bits Status"=w210:bool[], "Erro comunicação"=w213:bool)
              }
              frame True {
              }
            }
            "CUP_STAT" <- w105
            "CUP" <- w103
            n167 = case shown="False" "Case Constant\n(See Context Help)" {
              selector: "Case Constant\n(See Context Help)" -> [_ w204]
              tunnel: [w203 w204] -> w112
              tunnel: w111 -> [w202 _]
              tunnel: [w201 _] -> w113
              tunnel: [w200 _] -> w101
              tunnel: [w199 _] -> w104
              frame False {
                n168 = call "Get Status Controlador.vi"("Controlador"=w202) -> ("Status"=w199:string, "Parametros"=w201:string, "Bits Status"=w200:bool[], "Erro comunicação"=w203:bool)
              }
              frame True {
              }
            }
            "TUBO_STAT" <- w104
            "TUBO" <- w101
            n169 = case shown="False" "Case Constant\n(See Context Help)" {
              selector: "Case Constant\n(See Context Help)" -> [_ w254]
              tunnel: w123 -> [w253 _]
              tunnel: [w252 _] -> w94
              tunnel: [w251 _] -> w125
              tunnel: [w250 w254] -> w124
              tunnel: [w249 _] -> w107
              frame False {
                n170 = call "Get Status Controlador.vi"("Controlador"=w253) -> ("Status"=w249:string, "Parametros"=w251:string, "Bits Status"=w252:bool[], "Erro comunicação"=w250:bool)
              }
              frame True {
              }
            }
            "AH_STAT" <- w107
            "RA" <- w94
            n171 = stacked-sequence {
              frame #0 {
                # "Verifica se exite o arquivo da trapeira"
                # "Lê do arquivo qual o estado atual da trapeira"
                n172 = String To Path(string="C:\\TCS\\LOG\\SHUTTER\\SHUTTER.TXT" ("pathLogFocoString")) -> (path=w138:path)
                n173 = call <vilib>:"Check if File or Folder Exists.vi"("path"=w138) -> ("file or folder exists?"=w136:bool, "dup path"=w135:path)  [unwired: 8 in, 1 out]
                n174 = case shown="True" w136 {
                  tunnel: w135 -> [_ w148]
                  frame False {
                    n175 = local write "StatShutterFile"(" " ("StatShutterFile")) -> ()
                  }
                  frame True {
                    n176 = Open/Create/Replace File(file path (use dialog)=w148, operation (0:open)=T7."open", access (0:read/write)=enum16{"read/write", "read-only", "write-only"}."read/write") -> (refnum out=w145:refnum<file>, error out=w140:errorcluster)  [unwired: 3 in, 1 out]
                    n177 = Read from Text File(file (use dialog)=w145, error in=w140) -> (text=w144:string)  [unwired: 2 in, 3 out]
                    n178 = Match Pattern(string=w144, regular expression="SHUTTER") -> (after substring=w142:string)  [unwired: 1 in, 3 out]
                    n179 = call <vilib>:"Trim Whitespace.vi"("string"=w142) -> ("trimmed string"=w141:string)  [unwired: 1 in]
                    n180 = case shown="\"OPENED\", Default" w141 {
                      selector: w141 -> [w149 w150]
                      frame "OPENED", Default {
                        "StatShutterFile" <- w149
                      }
                      frame "CLOSED" {
                        n181 = local write "StatShutterFile"(w150) -> ()
                      }
                    }
                  }
                }
              }
              frame #1 {
                n182 = local read "timeStatShutterAlert"() -> (w153:i32)
                n183 = Tick Count (ms)() -> (millisecond timer value=w155:u32)
                n184 = Add(x=w153, y=3000) -> (x+y=w154:i32)
                n185 = Greater Or Equal?(x=w155, y=w154) -> (x >= y?=w151:bool)
                n186 = case shown="True" w151 {
                  frame False {
                  }
                  frame True {
                    n187 = local read "StatShutterFile"() -> (w157:string)
                    n188 = property on="LedShutter" class="Bool (strict)"() -> ("BoolText.Text"=w158:string)  [unwired: 2 in, 2 out]
                    n189 = Not Equal?(x=w158, y=w157) -> (x != y?=w156:bool)
                    n190 = case shown="False" w156 {
                      frame True {
                        n191 = property on="StatShutterFile" class="Str"("Blinking"=TRUE) -> ()  [unwired: 2 in, 2 out]
                      }
                      frame False {
                        n192 = property on="StatShutterFile" class="Str"("Blinking"=FALSE) -> ()  [unwired: 2 in, 2 out]
                      }
                    }
                  }
                }
              }
              frame #2 {
                n193 = disable-structure shown="Disabled" {
                  frame Disabled {
                    n194 = local read "StatShutterFile"() -> (w162:string)
                    n195 = property on="LedShutter" class="Bool (strict)"() -> ("BoolText.Text"=w163:string)  [unwired: 2 in, 2 out]
                    n196 = Not Equal?(x=w163, y=w162) -> (x != y?=w161:bool)
                    n197 = case shown="True" w161 {
                      frame False {
                        n198 = property on="Setup, Pointing & Guiding" class="TabCtl (strict)"() -> ("Pages"=w165:refnum<vi>[])  [unwired: 2 in, 2 out]
                        n199 = Index Array(array=w165, index=6) -> (element=w166:refnum<vi>)
                        n200 = property class="Page"(reference=w166, "FG Color"=u32 12369084) -> ()  [unwired: 1 in, 2 out]
                      }
                      frame True {
                        n201 = property on="Setup, Pointing & Guiding" class="TabCtl (strict)"() -> ("Pages"=w173:refnum<vi>[])  [unwired: 2 in, 2 out]
                        n202 = Index Array(array=w173, index=6) -> (element=w172:refnum<vi>)
                        n203 = property class="Page"(reference=w172) -> ("FG Color"=w169:u32)  [unwired: 1 in, 2 out]
                        n204 = Equal?(x=w169, y=u32 16711680) -> (x = y?=w168:bool)
                        n205 = case shown="False" w168 {
                          frame False {
                            n206 = property on="Setup, Pointing & Guiding" class="TabCtl (strict)"() -> ("Pages"=w175:refnum<vi>[])  [unwired: 2 in, 2 out]
                            n207 = Index Array(array=w175, index=6) -> (element=w176:refnum<vi>)
                            n208 = property class="Page"(reference=w176, "FG Color"=u32 16711680) -> ()  [unwired: 1 in, 2 out]
                          }
                          frame True {
                            n209 = property on="Setup, Pointing & Guiding" class="TabCtl (strict)"() -> ("Pages"=w179:refnum<vi>[])  [unwired: 2 in, 2 out]
                            n210 = Index Array(array=w179, index=6) -> (element=w180:refnum<vi>)
                            n211 = property class="Page"(reference=w180, "FG Color"=u32 12369084) -> ()  [unwired: 1 in, 2 out]
                          }
                        }
                      }
                    }
                  }
                  frame Enabled {
                  }
                }
              }
            }
            n212 = Index Array(array=w101, index=3) -> (element=w99:bool)
            n213 = call "Testa_Comunicação.vi"("DEC"=w93, "RA"=w94) -> ()  [unwired: 10 in]
            n214 = case shown="True" w99 {
              tunnel: ["S" "M"] -> w98
              frame False {
              }
              frame True {
              }
            }
            n215 = global write "Global_Telescopio.vi" "MOTOR LIGADO"(w98) -> ()
            n216 = case shown="False" w124 {
              tunnel: w94 -> [w241 _]
              tunnel: w125 -> [w240 _]
              tunnel: [w238 _] -> w110
              frame False {
                # "Leitura Válida"
                n217 = call <vilib>:"Trim Whitespace.vi"("string"=w240) -> ("trimmed string"=w238:string)  [unwired: 1 in]
                n218 = call "hms_rad.vi"("True = hora"=TRUE, "Texto Graus"=w238) -> ("radianos"=w235:dbl)  [unwired: 3 in]
                n219 = global write "Global_Telescopio.vi" "StatusAH"(w241) -> ()
                n220 = global read "Global_Telescopio.vi" "PosAH"() -> (w237:dbl)
                n221 = Equal?(x=w237, y=w235) -> (x = y?=w236:bool)
                n222 = case shown="False" w236 {
                  tunnel: w235 -> [w244 _]
                  frame False {
                    w243 = 0 ("CR AH")
                    n223 = local write "CR AH"(w243) -> ()
                    n224 = local write "CR AH UTILS"(w243) -> ()
                    n225 = global write "Global_Telescopio.vi" "PosAH"(w244) -> ()
                    "PosAH" <- w244
                    "Flag ativo AH" <- TRUE ("Flag ativo AH")
                  }
                  frame True {
                    n226 = local read "CR AH UTILS"() -> (w246:i32)
                    n227 = Increment(x=w246) -> (x+1=w245:i32)
                    n228 = local read "CR AH"() -> (w247:i32)
                    n229 = Increment(x=w247) -> (x+1=w248:i32)
                    n230 = local write "CR AH UTILS"(w245) -> ()
                    n231 = local write "CR AH"(w248) -> ()
                  }
                }
              }
              frame True {
                # "Erro na Leitura"
              }
            }
            "AH_ENC" <- w110
            n232 = case shown="False" w121 {
              tunnel: w122 -> [w226 _]
              tunnel: w93 -> [w225 _]
              tunnel: [w224 _] -> w109
              frame False {
                # "Leitura Válida"
                n233 = call <vilib>:"Trim Whitespace.vi"("string"=w226) -> ("trimmed string"=w224:string)  [unwired: 1 in]
                n234 = call "hms_rad.vi"("True = hora"=FALSE, "Texto Graus"=w224) -> ("radianos"=w221:dbl)  [unwired: 3 in]
                n235 = global write "Global_Telescopio.vi" "StatusDEC"(w225) -> ()
                n236 = global read "Global_Telescopio.vi" "PosDEC"() -> (w223:dbl)
                n237 = Equal?(x=w223, y=w221) -> (x = y?=w222:bool)
                n238 = case shown="False" w222 {
                  tunnel: w221 -> [w230 _]
                  frame False {
                    w229 = 0 ("CR DEC")
                    n239 = local write "CR DEC UTILS"(w229) -> ()
                    n240 = local write "CR DEC"(w229) -> ()
                    n241 = global write "Global_Telescopio.vi" "PosDEC"(w230) -> ()
                    "PosDEC" <- w230
                    "Flag ativo DEC" <- TRUE ("Flag ativo DEC")
                  }
                  frame True {
                    n242 = local read "CR DEC"() -> (w234:i32)
                    n243 = local read "CR DEC UTILS"() -> (w232:i32)
                    n244 = Increment(x=w232) -> (x+1=w231:i32)
                    n245 = Increment(x=w234) -> (x+1=w233:i32)
                    n246 = local write "CR DEC UTILS"(w231) -> ()
                    n247 = local write "CR DEC"(w233) -> ()
                  }
                }
              }
              frame True {
                # "Erro na Leitura"
              }
            }
            "DEC_ENC" <- w109
            n248 = case shown="False" w118 {
              tunnel: w103 -> [w208 _]
              tunnel: w117 -> [w207 _]
              tunnel: [w205 _] -> w108
              frame False {
                # "Leitura Válida"
                n249 = call <vilib>:"Trim Whitespace.vi"("string"=w207) -> ("trimmed string"=w205:string)  [unwired: 1 in]
                n250 = Decimal String To Number(string=w205) -> (number=w206:i32)  [unwired: 2 in, 1 out]
                n251 = global write "Global_Telescopio.vi" "StatusCUP"(w208) -> ()
                n252 = global write "Global_Telescopio.vi" "PosCUP"(w206) -> ()
              }
              frame True {
                # "Erro na Leitura"
              }
            }
            "DOMO_ENC" <- w108
            n253 = case shown="False" w112 {
              tunnel: w101 -> [w197 _]
              tunnel: w113 -> [w192 _]
              frame False {
                # "Leitura Válida"
                n254 = call <vilib>:"Trim Whitespace.vi"("string"=w192) -> ("trimmed string"=w196:string)  [unwired: 1 in]
                n255 = Decimal String To Number(string=w196) -> (number=w195:i32)  [unwired: 2 in, 1 out]
                n256 = global write "Global_Telescopio.vi" "StatusTUBO"(w197) -> ()
                n257 = global write "Global_Telescopio.vi" "PosFOCO"(w195) -> ()
                n258 = String Subset(string=w192, offset (0)=10, length (rest)=1 ("length (rest)")) -> (substring=→"EspAtual":string)
                n259 = Number To Decimal String(number=w195) -> (decimal integer string=w190:string)  [unwired: 1 in]
                "FOCO_ENC" <- w190
                n260 = Decimal String To Number(string=w190) -> (number=w188:i32)  [unwired: 2 in, 1 out]
                n261 = Greater Than 0?(x=w188) -> (x > 0?=w189:bool)
                n262 = case shown="True" w189 {
                  tunnel: w188 -> [_ w198]
                  frame False {
                  }
                  frame True {
                    n263 = global write "Global_Telescopio.vi" "Foco"(w198) -> ()
                  }
                }
              }
              frame True {
                # "Erro na Leitura"
              }
            }
            n264 = local read "shutterTimeOld"() -> (w92:i32)
            n265 = local read "sendCommandShutter"() -> (w87:bool)
            n266 = Tick Count (ms)() -> (millisecond timer value=w90:u32)
            n267 = Add(x=w92, y=40000) -> (x+y=w89:i32)
            n268 = Greater Or Equal?(x=w90, y=w89) -> (x >= y?=w88:bool)
            n269 = And(x=w88, y=w87) -> (x .and. y?=w86:bool)
            n270 = call "Sideral_Time.vi"("Fuso"=-3.0) -> ("TU"=→"UT":string, "Sideral Time"=w114:dbl)  [unwired: 2 in, 1 out]
            n271 = local read "LedPointing"() -> (w96:bool)
            n272 = case shown="True" w86 {
              frame False {
              }
              frame True {
                w182 = u16 4 items=["ZERO", "AH", "DEC", "TUBO", "CUP"] ("Controlador")
                # "Envia o comando para o controlador\nda cupula, após 40 segundos"
